vi "P4CMD Dialog_InitCtlsPrjOpts.vi"(7 "P4Proj UIDialog FP Refs":T1, 8 "error in (no error)":errorcluster, 10 "operation message":string, 11 "configuration data":string) -> (0 "error out":errorcluster)   [LabVIEW 2017, in "NI_SCC_P4CMD.lvlib"]
uses:
  <vilib>/SourceControl/Providers/P4CMD/NI_SCC_P4CMD.lvlib
  <vilib>/SourceControl/support/SCCSup ConfigData Conv.ctl
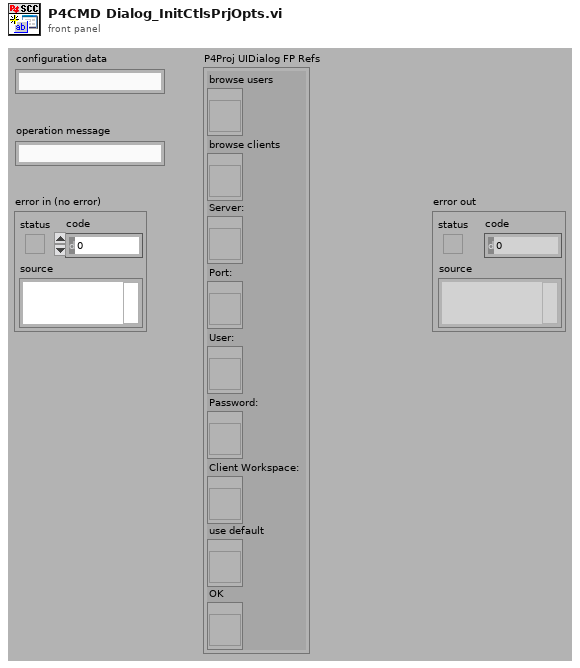
[diagram p1: front panel]
types:
  T1 = cluster{"browse users":refnum<vi>, "browse clients":refnum<vi>, "Server:":refnum<vi>, "Port:":refnum<vi>, "User:":refnum<vi>, "Password:":refnum<vi>, "Client Workspace:":refnum<vi>, "use default":refnum<vi>, "OK":refnum<vi>}
  T2 = typedef "SCCSup ConfigData Conv.ctl" = enum16{"from config data", "to config data"}
  T3 = typedef "NI_SCC_P4CMD.lvlib/P4CMD SCC Config Info.ctl" = cluster{"GBL lock on checkout?":bool, "GBL suppress dlgs?":bool, "port":string, "client":string, "user":string, "password":string}
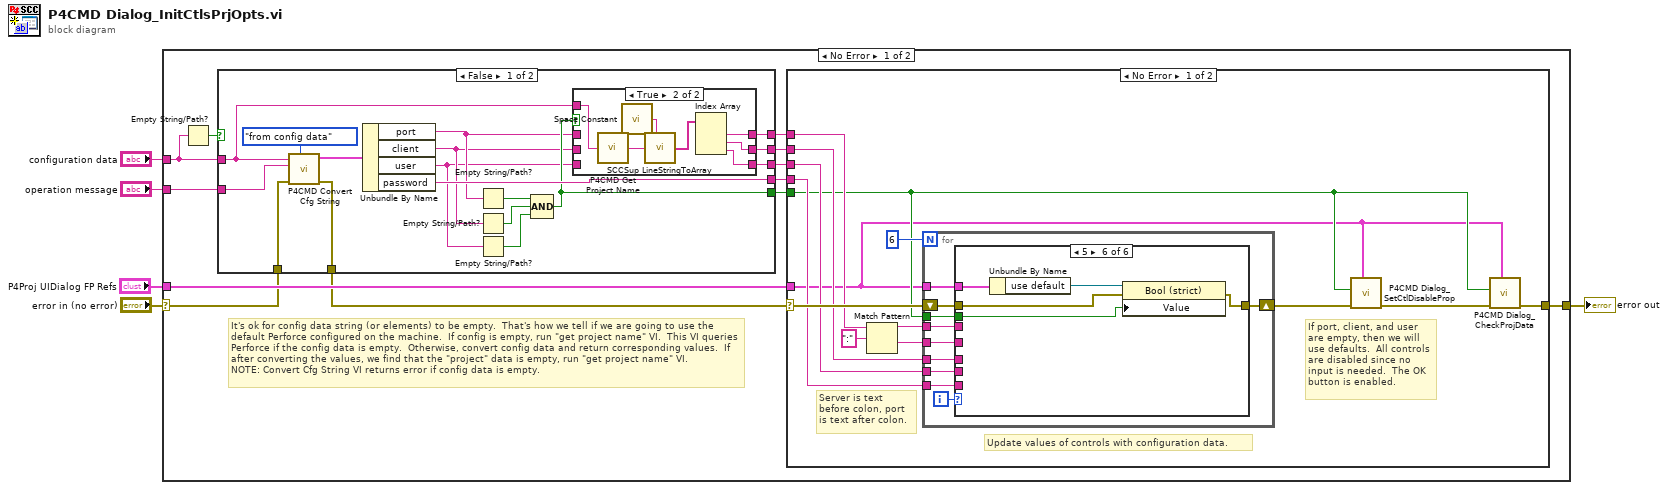
[diagram p0: block diagram]
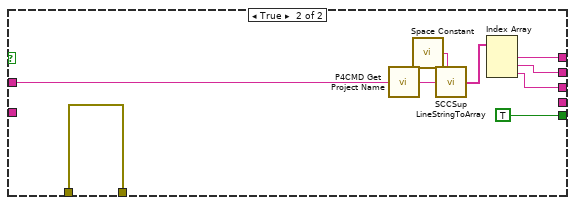
[diagram p3: hidden frame]
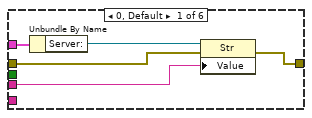
[diagram p4: hidden frame]
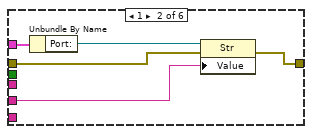
[diagram p5: hidden frame]
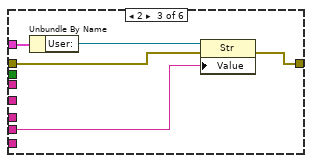
[diagram p6: hidden frame]
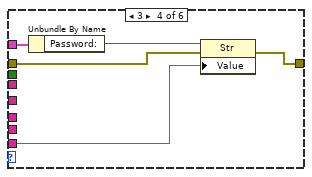
[diagram p7: hidden frame]
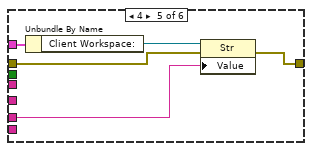
[diagram p8: hidden frame]
diagram:
  n1 = case shown="No Error" "error in (no error)" {
    selector: "error in (no error)" -> [w15 w109]
    tunnel: "P4Proj UIDialog FP Refs" -> [w17 _]
    tunnel: [w16 w109] -> w4
    tunnel: "configuration data" -> [w12 _]
    tunnel: "operation message" -> [w13 _]
    frame No Error {
      # "It's ok for config data string (or elements) to be empty.  That's how we tell if we are going to use the default Perforce configured on the machine.  If config is empty, run \"get project name\" VI.  This VI queries Perforce if the config data is empty.  Otherwise, convert config data and return corresponding values.  If after converting the values, we find that the \"project\" data is empty, run \"get project name\" VI.  \nNOTE: Convert Cfg String VI returns error if config data is empty."
      n2 = Empty String/Path?(string/path=w12) -> (empty?=w11:bool)
      n3 = case shown="False" w11 {
        tunnel: w15 -> [w33 w53]
        tunnel: [w32 w53] -> w14
        tunnel: w13 -> [w31 _]
        tunnel: w12 -> [w18 w52]
        tunnel: [w25 TRUE] -> w10
        tunnel: [w21 w47] -> w9
        tunnel: [w20 w46] -> w8
        tunnel: [w19 w45] -> w7
        tunnel: [w29 _] -> w6
        frame False {
          n4 = call <vilib>:"P4CMD Convert Cfg String.vi"("conversion action"=SCCSup_ConfigData_Conv."from config data", "error in (no error)"=w33, "operation message"=w31, "config data in"=w18) -> ("error out"=w32:errorcluster, "configuration details out"=w30:T3)  [unwired: 5 in, 1 out]
          n5 = Unbundle By Name(w30) -> ("port"=w24:string, "client"=w23:string, "user"=w22:string, "password"=w29:string)
          n6 = Empty String/Path?(string/path=w24) -> (empty?=w28:bool)
          n7 = Empty String/Path?(string/path=w23) -> (empty?=w27:bool)
          n8 = Empty String/Path?(string/path=w22) -> (empty?=w26:bool)
          n9 = Compound Arithmetic op=AND(w28, w27, w26) -> (w25:bool)
          n10 = case shown="True" w25 {
            tunnel: w24 -> [w37 _]
            tunnel: w23 -> [w36 _]
            tunnel: w22 -> [w35 _]
            tunnel: [w37 w40] -> w21
            tunnel: [w36 w39] -> w20
            tunnel: [w35 w38] -> w19
            tunnel: w18 -> [_ w41]
            frame False {
            }
            frame True {
              n11 = call <vilib>:"P4CMD Get Project Name.vi"("config data in"=w41) -> ("project name"=w44:string)  [unwired: 8 in]
              n12 = call <vilib>:"Space Constant.vi"() -> ("String"=w43:string)
              n13 = call <vilib>:"SCCSup LineStringToArray.vi"("delimiter (Tab)"=w43, "line string"=w44) -> ("line array"=w42:string[])  [unwired: 7 in]
              n14 = Index Array(array=w42) -> (element #1=w40:string, element #2=w39:string, element #3=w38:string)  [unwired: 3 in]
            }
          }
        }
        frame True {
          n15 = call <vilib>:"P4CMD Get Project Name.vi"("config data in"=w52) -> ("project name"=w50:string)  [unwired: 8 in]
          n16 = call <vilib>:"Space Constant.vi"() -> ("String"=w49:string)
          n17 = call <vilib>:"SCCSup LineStringToArray.vi"("delimiter (Tab)"=w49, "line string"=w50) -> ("line array"=w48:string[])  [unwired: 7 in]
          n18 = Index Array(array=w48) -> (element #1=w47:string, element #2=w46:string, element #3=w45:string)  [unwired: 3 in]
        }
      }
      n19 = case shown="No Error" w14 {
        selector: w14 -> [w60 w108]
        tunnel: w17 -> [w54 _]
        tunnel: [w61 w108] -> w16
        tunnel: w10 -> [w55 _]
        tunnel: w9 -> [w59 _]
        tunnel: w8 -> [w58 _]
        tunnel: w7 -> [w57 _]
        tunnel: w6 -> [w56 _]
        frame No Error {
          # "Update values of controls with configuration data."
          # "Server is text before colon, port is text after colon."
          # "If port, client, and user are empty, then we will use defaults.  All controls are disabled since no input is needed.  The OK button is enabled."
          n20 = Match Pattern(string=w59, regular expression=":" ("search string/char (-)")) -> (before substring=w65:string, after substring=w64:string)  [unwired: 1 in, 2 out]
          n21 = for {
            N: 6 -> [_]
            tunnel: w54 -> [w77]
            tunnel: w58 -> [w74]
            tunnel: w57 -> [w73]
            tunnel: w56 -> [w72]
            shift-right: [w71] -> w63
            shift-left: w60 -> [w75]
            tunnel: w65 -> [w70]
            tunnel: w64 -> [w69]
            tunnel: w55 -> [w68]
            i -> [w76]
            n22 = case shown="5" w76 {
              tunnel: w77 -> [w82 w87 w92 w97 w102 w107]
              tunnel: w75 -> [w80 w85 w90 w95 w100 w105]
              tunnel: w70 -> [w78 _ _ _ _ _]
              tunnel: w74 -> [_ _ _ _ w98 _]
              tunnel: w73 -> [_ _ w88 _ _ _]
              tunnel: w72 -> [_ _ _ w93 _ _]
              tunnel: [w79 w84 w89 w94 w99 w104] -> w71
              tunnel: w69 -> [_ w83 _ _ _ _]
              tunnel: w68 -> [_ _ _ _ _ w103]
              frame 0, Default {
                n23 = Unbundle By Name(w82) -> ("Server:"=w81:refnum<vi>)
                n24 = property class="Str"(reference=w81, error in=w80, "Value"=w78) -> (error out=w79:errorcluster)  [unwired: 1 out]
              }
              frame 1 {
                n25 = Unbundle By Name(w87) -> ("Port:"=w86:refnum<vi>)
                n26 = property class="Str"(reference=w86, error in=w85, "Value"=w83) -> (error out=w84:errorcluster)  [unwired: 1 out]
              }
              frame 2 {
                n27 = Unbundle By Name(w92) -> ("User:"=w91:refnum<vi>)
                n28 = property class="Str"(reference=w91, error in=w90, "Value"=w88) -> (error out=w89:errorcluster)  [unwired: 1 out]
              }
              frame 3 {
                n29 = Unbundle By Name(w97) -> ("Password:"=w96:refnum<vi>)
                n30 = property class="Str"(reference=w96, error in=w95, "Value"=w93) -> (error out=w94:errorcluster)  [unwired: 1 out]
              }
              frame 4 {
                n31 = Unbundle By Name(w102) -> ("Client Workspace:"=w101:refnum<vi>)
                n32 = property class="Str"(reference=w101, error in=w100, "Value"=w98) -> (error out=w99:errorcluster)  [unwired: 1 out]
              }
              frame 5 {
                n33 = Unbundle By Name(w107) -> ("use default"=w106:refnum<vi>)
                n34 = property class="Bool (strict)"(reference=w106, error in=w105, "Value"=w103) -> (error out=w104:errorcluster)  [unwired: 1 out]
              }
            }
          }
          n35 = call <vilib>:"P4CMD Dialog_SetCtlDisableProp.vi"("P4Proj UIDialog FP Refs"=w54, "error in (no error)"=w63, "use defaults?"=w55) -> ("error out"=w62:errorcluster)  [unwired: 8 in]
          n36 = call <vilib>:"P4CMD Dialog_CheckProjData.vi"("P4Proj UIDialog FP Refs"=w54, "error in (no error)"=w62, "use defaults? (F)"=w55) -> ("error out"=w61:errorcluster)  [unwired: 8 in]
        }
        frame Error {
        }
      }
    }
    frame Error {
    }
  }
  "error out" <- w4
